vi "KeyboardInput.vi"(0 "error in (no error)":errorcluster, 1 "Speed step":dbl, 2 "device ID":refnum<k1>) -> (3 "Control cluster":T1 {"Roll" scale=-1.0..1.0; "Pitch" scale=-1.0..1.0; "Vertical Speed" scale=-1.0..1.0; "Yaw Speed" scale=-1.0..1.0}, 4 "error out":errorcluster)   [LabVIEW 2014]
uses:
  <vilib>/Utility/inputDevices.llb/keyboardAcquire.vi
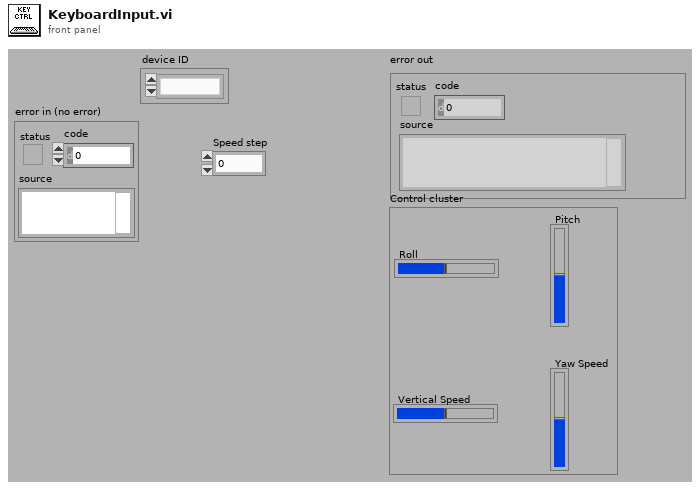
[diagram p1: front panel]
types:
  T1 = cluster{"Roll":dbl, "Pitch":dbl, "Vertical Speed":dbl, "Yaw Speed":dbl}
  T2 = enum16{"0", "1", "2", "3", "4", "5", "6", "7", "8", "9", "A", "B", "C", "D", "E", "F", "G", "H", "I", "J", "K", "L", "M", "N", "O", "P", "Q", "R", "S", "T", "U", "V", "W", "X", "Y", "Z", "F1", "F2", "F3", "F4", "F5", "F6", "F7", "F8", "F9", "F10", "F11", "F12", "F13", "F14", "F15", "ADD", "BACK", "BACKSLASH", "CAPITAL", "COMMA", "DECIMAL", "DELETE", "DIVIDE", "DOWN", "END", "EQUALS", "ESCAPE", "GRAVE (`)", "HOME", "INSERT", "LBRACKET", "LCONTROL", "LEFT", "L ALT", "LSHIFT", "LWIN", "MINUS", "MULTIPLY", "NEXT", "NUMLOCK", "NUMPAD_0", "NUMPAD_1", "NUMPAD_2", "NUMPAD_3", "NUMPAD_4", "NUMPAD_5", "NUMPAD_6", "NUMPAD_7", "NUMPAD_8", "NUMPAD_9", "PAUSE", "PERIOD", "PRIOR (PG UP)", "RBRACKET", "RCONTROL", "RETURN", "RIGHT", "R ALT", "RSHIFT", "RWIN", "SCROLL", "SEMICOLON", "SLASH", "SPACE", "SUBTRACT", "TAB", "UP", "ENTER (num pad)", "' (quote)"}[]
  T3 = enum16{"0", "1", "2", "3", "4", "5", "6", "7", "8", "9", "A", "B", "C", "D", "E", "F", "G", "H", "I", "J", "K", "L", "M", "N", "O", "P", "Q", "R", "S", "T", "U", "V", "W", "X", "Y", "Z", "F1", "F2", "F3", "F4", "F5", "F6", "F7", "F8", "F9", "F10", "F11", "F12", "F13", "F14", "F15", "ADD", "BACK", "BACKSLASH", "CAPITAL", "COMMA", "DECIMAL", "DELETE", "DIVIDE", "DOWN", "END", "EQUALS", "ESCAPE", "GRAVE (`)", "HOME", "INSERT", "LBRACKET", "LCONTROL", "LEFT", "L ALT", "LSHIFT", "LWIN", "MINUS", "MULTIPLY", "NEXT", "NUMLOCK", "NUMPAD_0", "NUMPAD_1", "NUMPAD_2", "NUMPAD_3", "NUMPAD_4", "NUMPAD_5", "NUMPAD_6", "NUMPAD_7", "NUMPAD_8", "NUMPAD_9", "PAUSE", "PERIOD", "PRIOR (PG UP)", "RBRACKET", "RCONTROL", "RETURN", "RIGHT", "R ALT", "RSHIFT", "RWIN", "SCROLL", "SEMICOLON", "SLASH", "SPACE", "SUBTRACT", "TAB", "UP", "ENTER (num pad)", "' (quote)"}
  T4 = cluster{dbl, dbl, "Speed step":dbl, "Speed step":dbl}
  T5 = cluster{dbl, "Speed step":dbl, "Speed step":dbl, dbl}
  T6 = cluster{"Speed step":dbl, dbl, "Speed step":dbl, dbl}
  T7 = cluster{dbl, "Speed step":dbl, dbl, "Speed step":dbl}
  T8 = cluster{"Speed step":dbl, dbl, dbl, "Speed step":dbl}
  T9 = cluster{"Speed step":dbl, "Speed step":dbl, dbl, dbl}
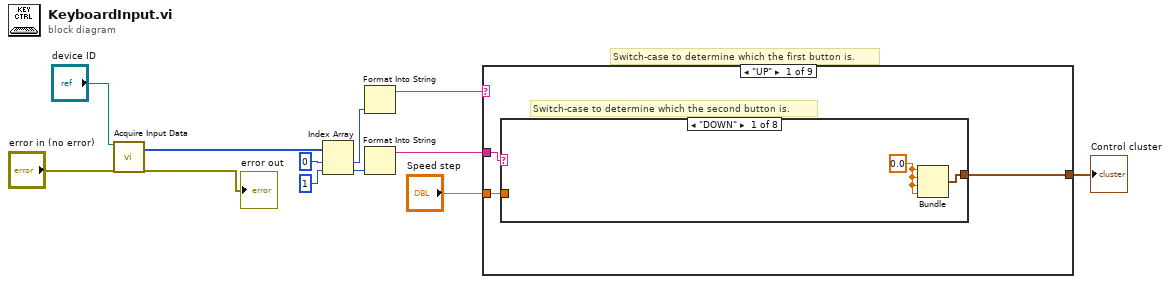
[diagram p0: block diagram]
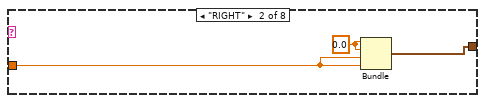
[diagram p2: hidden frame]
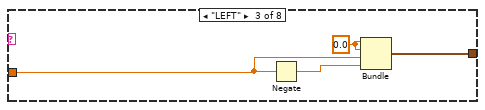
[diagram p3: hidden frame]
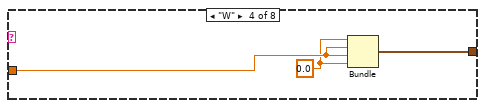
[diagram p4: hidden frame]
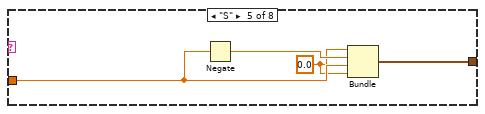
[diagram p5: hidden frame]
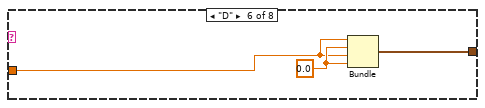
[diagram p6: hidden frame]
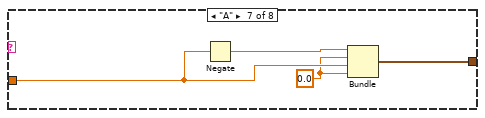
[diagram p7: hidden frame]
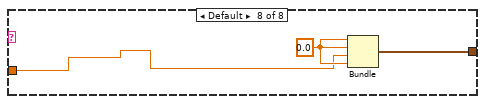
[diagram p8: hidden frame]
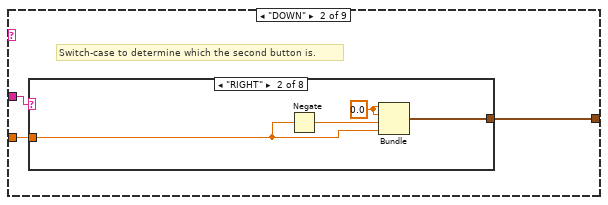
[diagram p9: hidden frame]
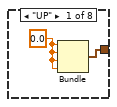
[diagram p10: hidden frame]
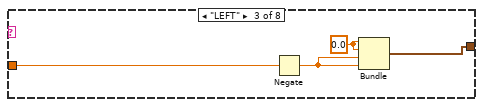
[diagram p11: hidden frame]
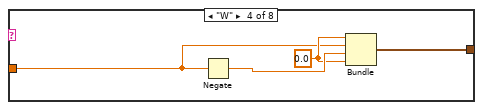
[diagram p12: hidden frame]
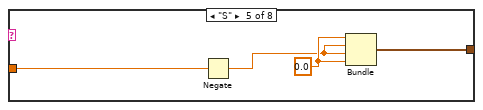
[diagram p13: hidden frame]
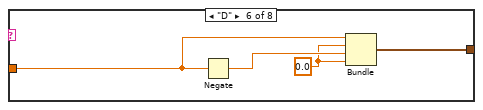
[diagram p14: hidden frame]
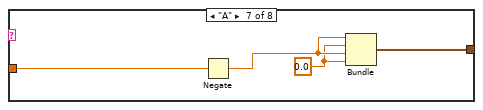
[diagram p15: hidden frame]
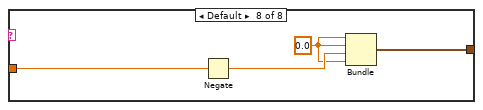
[diagram p16: hidden frame]
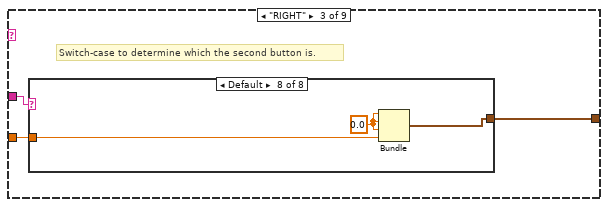
[diagram p17: hidden frame]
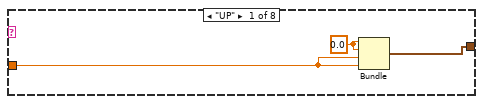
[diagram p18: hidden frame]
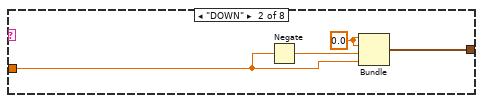
[diagram p19: hidden frame]
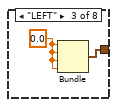
[diagram p20: hidden frame]
diagram:
  # "Switch-case to determine which the first button is."
  n1 = call-poly <vilib>:"Acquire Input Data.vi"("device ID"="device ID", "error in (no error)"="error in (no error)") -> ("keys pressed"=w6:T2, "error out"=→"error out":errorcluster)  [unwired: 15 in, 1 out]
  n2 = Index Array(array=w6, index #1=0, index #2=1) -> (element #1=w10:T3, element #2=w4:T3)
  n3 = Format Into String(w10) -> (resulting string=w12:string)  [unwired: 3 in, 1 out]
  n4 = Format Into String(w4) -> (resulting string=w3:string)  [unwired: 3 in, 1 out]
  n5 = case shown="\"UP\"" w12 {
    tunnel: w3 -> [w15 w43 w76 w106 w138 w167 w200 w229 _]
    tunnel: [w14 w42 w75 w104 w137 w166 w199 w228 w261] -> w1
    tunnel: "Speed step" -> [w13 w44 w77 w105 w139 w168 w201 w230 _]
    frame "UP" {
      # "Switch-case to determine which the second button is."
      n6 = case shown="\"DOWN\"" w15 {
        tunnel: [w16 w18 w24 w27 w30 w34 w37 w40] -> w14
        tunnel: w13 -> [_ w20 w23 w26 w31 w32 w38 w39]
        frame "DOWN" {
          w17 = 0.0
          n7 = Bundle(w17, w17, w17, w17) -> (w16:cluster{dbl, dbl, dbl, dbl})  [unwired: 1 in]
        }
        frame "RIGHT" {
          w19 = 0.0
          n8 = Bundle(w19, w19, "Speed step"=w20, "Speed step"=w20) -> (w18:T4)  [unwired: 1 in]
        }
        frame "LEFT" {
          w21 = 0.0
          n9 = Negate(x=w23) -> (-x=w22:dbl)
          n10 = Bundle(w21, w21, "Speed step"=w23, w22) -> (w24:cluster{dbl, dbl, "Speed step":dbl, dbl})  [unwired: 1 in]
        }
        frame "W" {
          w25 = 0.0
          n11 = Bundle(w25, "Speed step"=w26, "Speed step"=w26, w25) -> (w27:T5)  [unwired: 1 in]
        }
        frame "S" {
          w28 = 0.0
          n12 = Negate(x=w31) -> (-x=w29:dbl)
          n13 = Bundle(w28, w29, "Speed step"=w31, w28) -> (w30:cluster{dbl, dbl, "Speed step":dbl, dbl})  [unwired: 1 in]
        }
        frame "D" {
          w33 = 0.0
          n14 = Bundle("Speed step"=w32, w33, "Speed step"=w32, w33) -> (w34:T6)  [unwired: 1 in]
        }
        frame "A" {
          w35 = 0.0
          n15 = Negate(x=w38) -> (-x=w36:dbl)
          n16 = Bundle(w36, w35, "Speed step"=w38, w35) -> (w37:cluster{dbl, dbl, "Speed step":dbl, dbl})  [unwired: 1 in]
        }
        frame Default {
          w41 = 0.0
          n17 = Bundle(w41, w41, "Speed step"=w39, w41) -> (w40:cluster{dbl, dbl, "Speed step":dbl, dbl})  [unwired: 1 in]
        }
      }
    }
    frame "DOWN" {
      # "Switch-case to determine which the second button is."
      n18 = case shown="\"RIGHT\"" w43 {
        tunnel: [w46 w49 w54 w57 w61 w65 w69 w71] -> w42
        tunnel: w44 -> [_ w47 w53 w55 w62 w64 w70 w74]
        frame "UP" {
          w45 = 0.0
          n19 = Bundle(w45, w45, w45, w45) -> (w46:cluster{dbl, dbl, dbl, dbl})  [unwired: 1 in]
        }
        frame "RIGHT" {
          w48 = 0.0
          n20 = Negate(x=w47) -> (-x=w50:dbl)
          n21 = Bundle(w48, w48, w50, "Speed step"=w47) -> (w49:cluster{dbl, dbl, dbl, "Speed step":dbl})  [unwired: 1 in]
        }
        frame "LEFT" {
          w52 = 0.0
          n22 = Negate(x=w53) -> (-x=w51:dbl)
          n23 = Bundle(w52, w52, w51, w51) -> (w54:cluster{dbl, dbl, dbl, dbl})  [unwired: 1 in]
        }
        frame "W" {
          w56 = 0.0
          n24 = Negate(x=w55) -> (-x=w58:dbl)
          n25 = Bundle(w56, "Speed step"=w55, w58, w56) -> (w57:cluster{dbl, "Speed step":dbl, dbl, dbl})  [unwired: 1 in]
        }
        frame "S" {
          w60 = 0.0
          n26 = Negate(x=w62) -> (-x=w59:dbl)
          n27 = Bundle(w60, w59, w59, w60) -> (w61:cluster{dbl, dbl, dbl, dbl})  [unwired: 1 in]
        }
        frame "D" {
          w63 = 0.0
          n28 = Negate(x=w64) -> (-x=w66:dbl)
          n29 = Bundle("Speed step"=w64, w63, w66, w63) -> (w65:cluster{"Speed step":dbl, dbl, dbl, dbl})  [unwired: 1 in]
        }
        frame "A" {
          w67 = 0.0
          n30 = Negate(x=w70) -> (-x=w68:dbl)
          n31 = Bundle(w68, w67, w68, w67) -> (w69:cluster{dbl, dbl, dbl, dbl})  [unwired: 1 in]
        }
        frame Default {
          w72 = 0.0
          n32 = Negate(x=w74) -> (-x=w73:dbl)
          n33 = Bundle(w72, w72, w73, w72) -> (w71:cluster{dbl, dbl, dbl, dbl})  [unwired: 1 in]
        }
      }
    }
    frame "RIGHT" {
      # "Switch-case to determine which the second button is."
      n34 = case shown="Default" w76 {
        tunnel: [w78 w81 w85 w89 w92 w96 w99 w101] -> w75
        tunnel: w77 -> [w80 w84 _ w87 w93 w95 w100 w103]
        frame "UP" {
          w79 = 0.0
          n35 = Bundle(w79, w79, "Speed step"=w80, "Speed step"=w80) -> (w78:T4)  [unwired: 1 in]
        }
        frame "DOWN" {
          w82 = 0.0
          n36 = Negate(x=w84) -> (-x=w83:dbl)
          n37 = Bundle(w82, w82, w83, "Speed step"=w84) -> (w81:cluster{dbl, dbl, dbl, "Speed step":dbl})  [unwired: 1 in]
        }
        frame "LEFT" {
          w86 = 0.0
          n38 = Bundle(w86, w86, w86, w86) -> (w85:cluster{dbl, dbl, dbl, dbl})  [unwired: 1 in]
        }
        frame "W" {
          w88 = 0.0
          n39 = Bundle(w88, "Speed step"=w87, w88, "Speed step"=w87) -> (w89:T7)  [unwired: 1 in]
        }
        frame "S" {
          w91 = 0.0
          n40 = Negate(x=w93) -> (-x=w90:dbl)
          n41 = Bundle(w91, w90, w91, "Speed step"=w93) -> (w92:cluster{dbl, dbl, dbl, "Speed step":dbl})  [unwired: 1 in]
        }
        frame "D" {
          w94 = 0.0
          n42 = Bundle("Speed step"=w95, w94, w94, "Speed step"=w95) -> (w96:T8)  [unwired: 1 in]
        }
        frame "A" {
          w97 = 0.0
          n43 = Negate(x=w100) -> (-x=w98:dbl)
          n44 = Bundle(w98, w97, w97, "Speed step"=w100) -> (w99:cluster{dbl, dbl, dbl, "Speed step":dbl})  [unwired: 1 in]
        }
        frame Default {
          w102 = 0.0
          n45 = Bundle(w102, w102, w102, "Speed step"=w103) -> (w101:cluster{dbl, dbl, dbl, "Speed step":dbl})  [unwired: 1 in]
        }
      }
    }
    frame "LEFT" {
      # "Switch-case to determine which the second button is."
      n46 = case shown="\"A\"" w106 {
        tunnel: [w107 w111 w115 w119 w123 w127 w131 w136] -> w104
        tunnel: w105 -> [w109 w114 _ w118 w124 w126 w132 w134]
        frame "UP" {
          w108 = 0.0
          n47 = Negate(x=w109) -> (-x=w110:dbl)
          n48 = Bundle(w108, w108, "Speed step"=w109, w110) -> (w107:cluster{dbl, dbl, "Speed step":dbl, dbl})  [unwired: 1 in]
        }
        frame "DOWN" {
          w112 = 0.0
          n49 = Negate(x=w114) -> (-x=w113:dbl)
          n50 = Bundle(w112, w112, w113, w113) -> (w111:cluster{dbl, dbl, dbl, dbl})  [unwired: 1 in]
        }
        frame "RIGHT" {
          w116 = 0.0
          n51 = Bundle(w116, w116, w116, w116) -> (w115:cluster{dbl, dbl, dbl, dbl})  [unwired: 1 in]
        }
        frame "W" {
          w117 = 0.0
          n52 = Negate(x=w118) -> (-x=w120:dbl)
          n53 = Bundle(w117, "Speed step"=w118, w117, w120) -> (w119:cluster{dbl, "Speed step":dbl, dbl, dbl})  [unwired: 1 in]
        }
        frame "S" {
          w122 = 0.0
          n54 = Negate(x=w124) -> (-x=w121:dbl)
          n55 = Bundle(w122, w121, w122, w121) -> (w123:cluster{dbl, dbl, dbl, dbl})  [unwired: 1 in]
        }
        frame "D" {
          w125 = 0.0
          n56 = Negate(x=w126) -> (-x=w128:dbl)
          n57 = Bundle("Speed step"=w126, w125, w125, w128) -> (w127:cluster{"Speed step":dbl, dbl, dbl, dbl})  [unwired: 1 in]
        }
        frame "A" {
          w129 = 0.0
          n58 = Negate(x=w132) -> (-x=w130:dbl)
          n59 = Bundle(w130, w129, w129, w130) -> (w131:cluster{dbl, dbl, dbl, dbl})  [unwired: 1 in]
        }
        frame Default {
          w135 = 0.0
          n60 = Negate(x=w134) -> (-x=w133:dbl)
          n61 = Bundle(w135, w135, w135, w133) -> (w136:cluster{dbl, dbl, dbl, dbl})  [unwired: 1 in]
        }
      }
    }
    frame "W" {
      # "Switch-case to determine which the second button is."
      n62 = case shown="Default" w138 {
        tunnel: [w140 w143 w147 w150 w154 w156 w161 w165] -> w137
        tunnel: w139 -> [w142 w146 w149 w153 _ w158 w160 w164]
        frame "UP" {
          w141 = 0.0
          n63 = Negate(x=w142) -> ()  [unwired: 1 out]
          n64 = Bundle("Speed step"=w142, w141, "Speed step"=w142, w141) -> (w140:T6)  [unwired: 1 in]
        }
        frame "DOWN" {
          w144 = 0.0
          n65 = Negate(x=w146) -> (-x=w145:dbl)
          n66 = Bundle("Speed step"=w146, w144, w145, w144) -> (w143:cluster{"Speed step":dbl, dbl, dbl, dbl})  [unwired: 1 in]
        }
        frame "RIGHT" {
          w148 = 0.0
          n67 = Bundle("Speed step"=w149, w148, w148, "Speed step"=w149) -> (w147:T8)  [unwired: 1 in]
        }
        frame "LEFT" {
          w151 = 0.0
          n68 = Negate(x=w153) -> (-x=w152:dbl)
          n69 = Bundle("Speed step"=w153, w151, w151, w152) -> (w150:cluster{"Speed step":dbl, dbl, dbl, dbl})  [unwired: 1 in]
        }
        frame "S" {
          w155 = 0.0
          n70 = Bundle(w155, w155, w155, w155) -> (w154:cluster{dbl, dbl, dbl, dbl})  [unwired: 1 in]
        }
        frame "D" {
          w157 = 0.0
          n71 = Bundle("Speed step"=w158, "Speed step"=w158, w157, w157) -> (w156:T9)  [unwired: 1 in]
        }
        frame "A" {
          w162 = 0.0
          n72 = Negate(x=w160) -> (-x=w159:dbl)
          n73 = Bundle(w159, "Speed step"=w160, w162, w162) -> (w161:cluster{dbl, "Speed step":dbl, dbl, dbl})  [unwired: 1 in]
        }
        frame Default {
          w163 = 0.0
          n74 = Bundle(w163, "Speed step"=w164, w163, w163) -> (w165:cluster{dbl, "Speed step":dbl, dbl, dbl})  [unwired: 1 in]
        }
      }
    }
    frame "S" {
      # "Switch-case to determine which the second button is."
      n75 = case shown="Default" w167 {
        tunnel: [w169 w173 w177 w181 w185 w189 w191 w197] -> w166
        tunnel: w168 -> [w171 w176 w179 w184 _ w188 w194 w198]
        frame "UP" {
          w170 = 0.0
          n76 = Negate(x=w171) -> (-x=w172:dbl)
          n77 = Bundle(w172, w170, "Speed step"=w171, w170) -> (w169:cluster{dbl, dbl, "Speed step":dbl, dbl})  [unwired: 1 in]
        }
        frame "DOWN" {
          w174 = 0.0
          n78 = Negate(x=w176) -> (-x=w175:dbl)
          n79 = Bundle(w175, w174, w175, w174) -> (w173:cluster{dbl, dbl, dbl, dbl})  [unwired: 1 in]
        }
        frame "RIGHT" {
          w178 = 0.0
          n80 = Negate(x=w179) -> (-x=w180:dbl)
          n81 = Bundle(w180, w178, w178, "Speed step"=w179) -> (w177:cluster{dbl, dbl, dbl, "Speed step":dbl})  [unwired: 1 in]
        }
        frame "LEFT" {
          w182 = 0.0
          n82 = Negate(x=w184) -> (-x=w183:dbl)
          n83 = Bundle(w183, w182, w182, w183) -> (w181:cluster{dbl, dbl, dbl, dbl})  [unwired: 1 in]
        }
        frame "W" {
          w186 = 0.0
          n84 = Bundle(w186, w186, w186, w186) -> (w185:cluster{dbl, dbl, dbl, dbl})  [unwired: 1 in]
        }
        frame "D" {
          w190 = 0.0
          n85 = Negate(x=w188) -> (-x=w187:dbl)
          n86 = Bundle("Speed step"=w188, w187, w190, w190) -> (w189:cluster{"Speed step":dbl, dbl, dbl, dbl})  [unwired: 1 in]
        }
        frame "A" {
          w192 = 0.0
          n87 = Negate(x=w194) -> (-x=w193:dbl)
          n88 = Bundle(w193, w193, w192, w192) -> (w191:cluster{dbl, dbl, dbl, dbl})  [unwired: 1 in]
        }
        frame Default {
          w195 = 0.0
          n89 = Negate(x=w198) -> (-x=w196:dbl)
          n90 = Bundle(w195, w196, w195, w195) -> (w197:cluster{dbl, dbl, dbl, dbl})  [unwired: 1 in]
        }
      }
    }
    frame "D" {
      # "Switch-case to determine which the second button is."
      n91 = case shown="Default" w200 {
        tunnel: [w202 w205 w209 w212 w216 w221 w223 w227] -> w199
        tunnel: w201 -> [w204 w208 w211 w215 w218 w220 _ w226]
        frame "UP" {
          w203 = 0.0
          n92 = Bundle(w203, "Speed step"=w204, "Speed step"=w204, w203) -> (w202:T5)  [unwired: 1 in]
        }
        frame "DOWN" {
          w206 = 0.0
          n93 = Negate(x=w208) -> (-x=w207:dbl)
          n94 = Bundle(w206, "Speed step"=w208, w207, w206) -> (w205:cluster{dbl, "Speed step":dbl, dbl, dbl})  [unwired: 1 in]
        }
        frame "RIGHT" {
          w210 = 0.0
          n95 = Bundle(w210, "Speed step"=w211, w210, "Speed step"=w211) -> (w209:T7)  [unwired: 1 in]
        }
        frame "LEFT" {
          w213 = 0.0
          n96 = Negate(x=w215) -> (-x=w214:dbl)
          n97 = Bundle(w213, "Speed step"=w215, w213, w214) -> (w212:cluster{dbl, "Speed step":dbl, dbl, dbl})  [unwired: 1 in]
        }
        frame "W" {
          w217 = 0.0
          n98 = Bundle("Speed step"=w218, "Speed step"=w218, w217, w217) -> (w216:T9)  [unwired: 1 in]
        }
        frame "S" {
          w222 = 0.0
          n99 = Negate(x=w220) -> (-x=w219:dbl)
          n100 = Bundle("Speed step"=w220, w219, w222, w222) -> (w221:cluster{"Speed step":dbl, dbl, dbl, dbl})  [unwired: 1 in]
        }
        frame "A" {
          w224 = 0.0
          n101 = Bundle(w224, w224, w224, w224) -> (w223:cluster{dbl, dbl, dbl, dbl})  [unwired: 1 in]
        }
        frame Default {
          w225 = 0.0
          n102 = Bundle("Speed step"=w226, w225, w225, w225) -> (w227:cluster{"Speed step":dbl, dbl, dbl, dbl})  [unwired: 1 in]
        }
      }
    }
    frame "A" {
      # "Switch-case to determine which the second button is."
      n103 = case shown="Default" w229 {
        tunnel: [w231 w235 w239 w243 w249 w251 w255 w259] -> w228
        tunnel: w230 -> [w233 w238 w241 w246 w247 w254 _ w260]
        frame "UP" {
          w232 = 0.0
          n104 = Negate(x=w233) -> (-x=w234:dbl)
          n105 = Bundle(w232, w234, "Speed step"=w233, w232) -> (w231:cluster{dbl, dbl, "Speed step":dbl, dbl})  [unwired: 1 in]
        }
        frame "DOWN" {
          w236 = 0.0
          n106 = Negate(x=w238) -> (-x=w237:dbl)
          n107 = Bundle(w236, w237, w237, w236) -> (w235:cluster{dbl, dbl, dbl, dbl})  [unwired: 1 in]
        }
        frame "RIGHT" {
          w240 = 0.0
          n108 = Negate(x=w241) -> (-x=w242:dbl)
          n109 = Bundle(w240, w242, w240, "Speed step"=w241) -> (w239:cluster{dbl, dbl, dbl, "Speed step":dbl})  [unwired: 1 in]
        }
        frame "LEFT" {
          w244 = 0.0
          n110 = Negate(x=w246) -> (-x=w245:dbl)
          n111 = Bundle(w244, w245, w244, w245) -> (w243:cluster{dbl, dbl, dbl, dbl})  [unwired: 1 in]
        }
        frame "W" {
          w250 = 0.0
          n112 = Negate(x=w247) -> (-x=w248:dbl)
          n113 = Bundle(w248, "Speed step"=w247, w250, w250) -> (w249:cluster{dbl, "Speed step":dbl, dbl, dbl})  [unwired: 1 in]
        }
        frame "S" {
          w252 = 0.0
          n114 = Negate(x=w254) -> (-x=w253:dbl)
          n115 = Bundle(w253, w253, w252, w252) -> (w251:cluster{dbl, dbl, dbl, dbl})  [unwired: 1 in]
        }
        frame "D" {
          w256 = 0.0
          n116 = Bundle(w256, w256, w256, w256) -> (w255:cluster{dbl, dbl, dbl, dbl})  [unwired: 1 in]
        }
        frame Default {
          w257 = 0.0
          n117 = Negate(x=w260) -> (-x=w258:dbl)
          n118 = Bundle(w258, w257, w257, w257) -> (w259:cluster{dbl, dbl, dbl, dbl})  [unwired: 1 in]
        }
      }
    }
    frame Default {
      w262 = 0.0
      n119 = Bundle(w262, w262, w262, w262) -> (w261:cluster{dbl, dbl, dbl, dbl})  [unwired: 1 in]
    }
  }
  "Control cluster" <- w1
